vi "Pattern File List.vi"(8 "error in (no error)":errorcluster) -> (0 "error out":errorcluster, 3 "Pattern Paths":path[](array[path]))   [LabVIEW 2013]
uses:
  HHMI - Filepaths global.vi
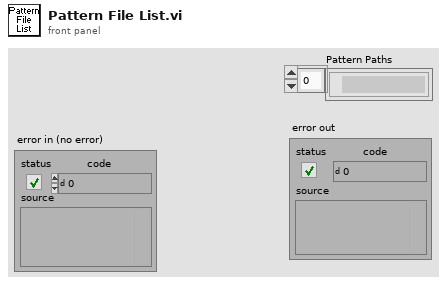
[diagram p1: front panel]
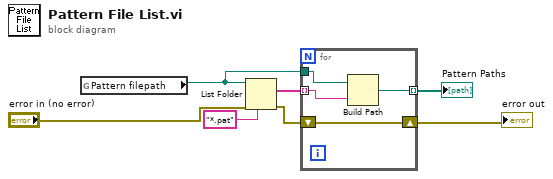
[diagram p0: block diagram]
diagram:
  n1 = global read "HHMI - Filepaths global.vi" "Pattern filepath"() -> (w5:path)
  n2 = List Folder(path=w5, pattern="*.pat", error in="error in (no error)") -> (filenames=w6:string[], error out=w2:errorcluster)  [unwired: 1 in, 2 out]
  n3 = for {
    tunnel: w6 -> [w10] mode=indexing
    tunnel: w5 -> [w11]
    tunnel: [w9] -> w4 mode=indexing
    shift-right: [w8] -> w1
    shift-left: w2 -> [w8]
    n4 = Build Path(base path=w11, name or relative path=w10) -> (appended path=w9:path)
  }
  "Pattern Paths" <- w4
  "error out" <- w1
